vi "Write U32.vi"(0 "I2C In":refnum<class "I2C.lvclass">, 1 "Slave Address":u8, 5 "Register":u32, 7 "Value":u32, 11 "Error In":errorcluster, 12 "Register Size":T2, 13 "Byte Order":T1) -> (4 "I2C Out":refnum<class "I2C.lvclass">, 15 "Error Out":errorcluster)   [LabVIEW 2020, in "lv_i2c_hal.lvlib" / "I2C.lvclass"]
uses:
  I2C.lvclass
  Register Address Size.ctl
  Byte Order.ctl
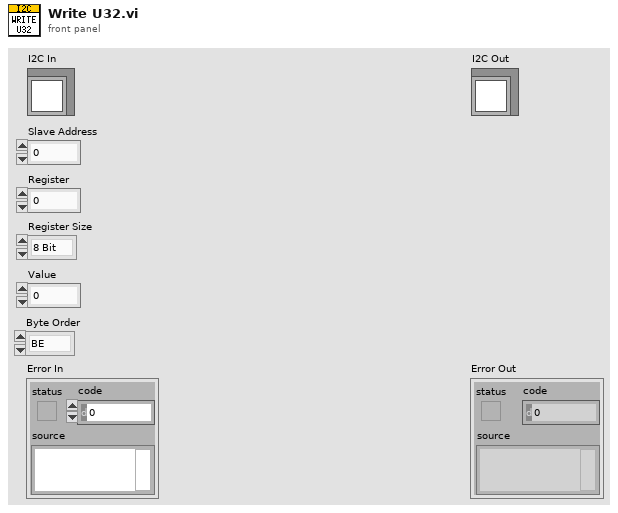
[diagram p1: front panel]
types:
  T1 = typedef "lv_i2c_hal.lvlib/I2C.lvclass/Byte Order.ctl" = enum16{"BE", "LE"}
  T2 = typedef "lv_i2c_hal.lvlib/I2C.lvclass/Register Address Size.ctl" = enum16{"8 Bit", "16 Bit", "24 Bit", "32 Bit"}
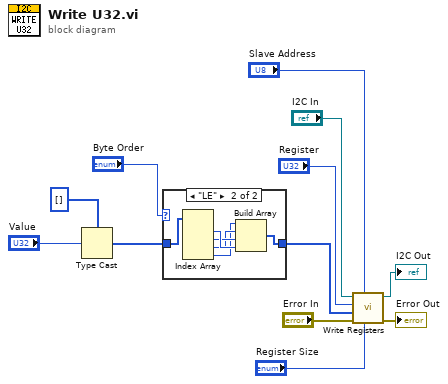
[diagram p0: block diagram]
diagram:
  n1 = Type Cast(type=u8[] [], x="Value") -> (*(type *) &x=w6:u8[])
  n2 = case shown="\"LE\"" "Byte Order" {
    tunnel: [w13 w18] -> w5
    tunnel: w6 -> [w13 w19]
    frame "BE", Default {
    }
    frame "LE" {
      n3 = Index Array(array=w19) -> (element #1=w17:u8, element #2=w16:u8, element #3=w15:u8, element #4=w14:u8)  [unwired: 4 in]
      n4 = Build Array(w14, w15, w16, w17) -> (w18:u8[])
    }
  }
  n5 = call "Write Registers.vi"("Register Size"="Register Size", "Slave Address"="Slave Address", "Error In"="Error In", "Values"=w5, "Register"="Register", "I2C In"="I2C In") -> ("Error Out"=→"Error Out":errorcluster, "I2C Out"=→"I2C Out":refnum<class "I2C.lvclass">)  [unwired: 4 in]
